vi "EN50160 Aggregation (3s, 10s, 10min).vi"(0 "half-cycle frequency":T4, 1 "voltage RMS values":dbl[](array[numeric]), 2 "fundamental voltage unbalance u2 [%]":dbl, 3 "signaling voltage RMS values":dbl[](array[numeric]), 4 "system info in":refnum<class "EP System Info.lvclass">, 5 "error in (no error)":errorcluster, 6 "reset? (F)":bool, 7 "voltage THD [%]":dbl[](array[numeric]), 8 "data timestamp":timestamp, 9 "harmonic subgroups complex spectra":cluster{"f0":dbl, "df":dbl, "vectors":cdb[]}[](array[cluster]), 11 "voltage flags? (F)":bool[](array[boolean])) -> (14 "10min values":T3, 15 "10s values":T2, 16 "3s values":T1, 18 "system info out":refnum<class "EP System Info.lvclass">, 19 "error out":errorcluster)   [LabVIEW 2014, in "NI_EP_Power Quality.lvlib"]
doc: "Calculates aggregated values of power quality parameters for specific intervals. You use the aggregated values for further evaluations according to EN 50160:2007. The aggregation methods are compliant with Class S in IEC 61000-4-30:2008. The aggregation is based on a 10-cycle time interval for a 50 Hz power system or 12-cycle time interval for a 60 Hz power system. There is no overlap between aggregation intervals. This VI automatically restarts accumulation at the beginning of the next 10/12-cycle time interval after the previous interval expires. You must manually select the polymorphic instance you want to use.\n\nThis VI supports measuring single-bus single-line or multiple-bus single-line systems."
uses:
  <vilib>/addons/Electrical Power/PQ/NI_EP_Power Quality.lvlib
  <vilib>/addons/Electrical Power/PQ/Common/Classes/System Info/EP System Info.lvclass
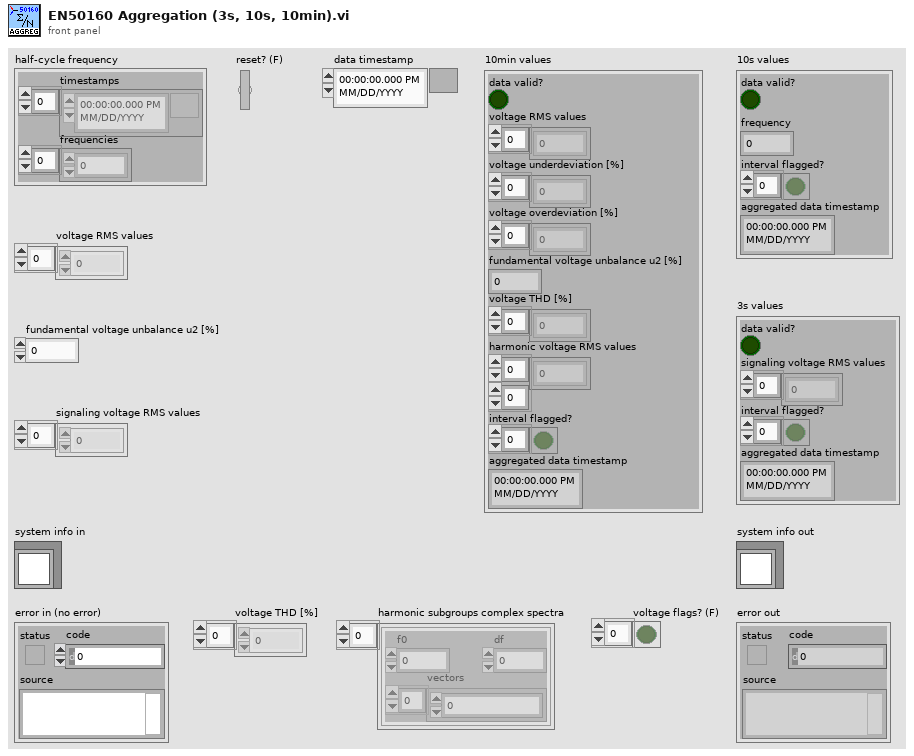
[diagram p1: front panel]
types:
  T1 = cluster{"data valid?":bool, "signaling voltage RMS values":dbl[], "interval flagged?":bool[], "aggregated data timestamp":timestamp}
  T2 = cluster{"data valid?":bool, "frequency":dbl, "interval flagged?":bool[], "aggregated data timestamp":timestamp}
  T3 = cluster{"data valid?":bool, "voltage RMS values":dbl[], "voltage underdeviation [%]":dbl[], "voltage overdeviation [%]":dbl[], "fundamental voltage unbalance u2 [%] ":dbl, "voltage THD [%]":dbl[], "harmonic voltage RMS values":dbl[][], "interval flagged?":bool[], "aggregated data timestamp":timestamp}
  T4 = cluster{"timestamps":timestamp[], "frequencies":dbl[]}
  T5 = cluster{"data valid?":bool, "voltage RMS values":dbl[], "voltage underdeviation [%]":dbl[], "voltage overdeviation [%]":dbl[], "fundamental voltage unbalance u2 [%]  ":dbl, "voltage THD [%]":dbl[], "harmonic voltage RMS values":dbl[][], "interval flagged?":bool[], "aggregated data timestamp":timestamp}
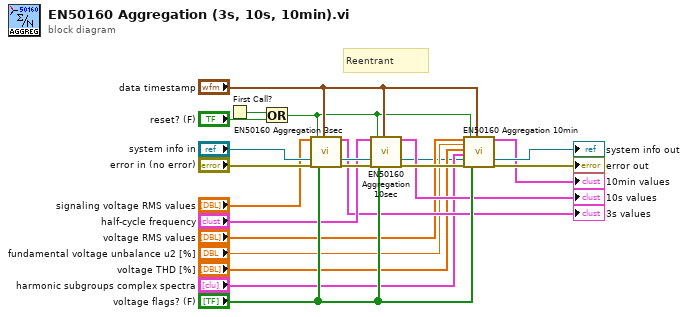
[diagram p0: block diagram]
diagram:
  # "Reentrant"
  n1 = First Call?() -> (First Call?: T/F=w3:bool)
  n2 = Or(x=w3, y="reset? (F)") -> (x .or. y?=w1:bool)
  n3 = call <vilib>:"EN50160 Aggregation 3sec.vi"("signaling voltage RMS values"="signaling voltage RMS values", "system info in"="system info in", "error in (no error)"="error in (no error)", "reset? (F)"=w1, "voltage flags? (F)"="voltage flags? (F)", "data timestamp"="data timestamp") -> ("3s values"=→"3s values":T1, "system info out"=w15:refnum<class "EP System Info.lvclass">, "error out"=w20:errorcluster)  [unwired: 11 in]
  n4 = call <vilib>:"EN50160 Aggregation 10sec.vi"("half-cycle frequency"="half-cycle frequency", "system info in"=w15, "error in (no error)"=w20, "reset? (F)"=w1, "voltage flags? (F)"="voltage flags? (F)", "data timestamp"="data timestamp") -> ("10s values"=→"10s values":T2, "system info out"=w4:refnum<class "EP System Info.lvclass">, "error out"=w21:errorcluster)  [unwired: 11 in]
  n5 = call <vilib>:"EN50160 Aggregation 10min.vi"("voltage RMS values"="voltage RMS values", "fundamental voltage unbalance u2 [%]"="fundamental voltage unbalance u2 [%]", "voltage THD [%]"="voltage THD [%]", "harmonic subgroups complex spectra"="harmonic subgroups complex spectra", "system info in"=w4, "error in (no error)"=w21, "reset? (F)"=w1, "voltage flags? (F)"="voltage flags? (F)", "data timestamp"="data timestamp") -> ("10min values"=→"10min values":T5, "system info out"=→"system info out":refnum<class "EP System Info.lvclass">, "error out"=→"error out":errorcluster)  [unwired: 8 in]
